vi "Write AcknowledgeMsg.vi"(8 "error in (no error)":errorcluster, 10 "AcknowledgeMsg.lvlib:AcknowledgeMsg.lvclass":refnum<class "CS++AcknowledgeMsg.lvclass">, 11 "AsynchReturnMsg in":refnum<class "CS++AsynchReturnMsg.lvclass">) -> (0 "error out":errorcluster, 3 "AsynchReturnMsg out":refnum<class "CS++AsynchReturnMsg.lvclass">)   [LabVIEW 2016, in "CS++AsynchReturnMsg.lvlib" / "CS++AsynchReturnMsg.lvclass"]
uses:
  CS++AsynchReturnMsg.lvclass
  CS++AcknowledgeMsg/CS++AcknowledgeMsg.lvclass
  CS++AsynchReturnMsg.lvclass/CS++AsynchReturnMsg.ctl
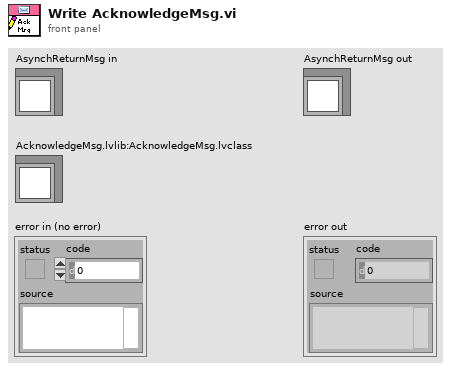
[diagram p1: front panel]
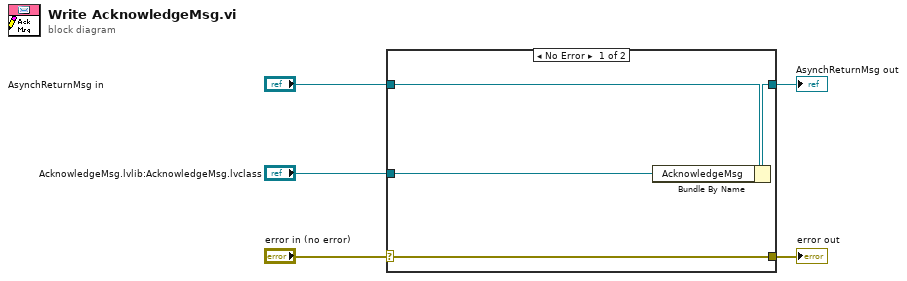
[diagram p0: block diagram]
diagram:
  n1 = case shown="No Error" "error in (no error)" {
    selector: "error in (no error)" -> [w9 w10]
    tunnel: [w9 w10] -> w4
    tunnel: [w7 w11] -> w2
    tunnel: "AsynchReturnMsg in" -> [w8 w11]
    tunnel: "AcknowledgeMsg.lvlib:AcknowledgeMsg.lvclass" -> [w6 _]
    frame No Error {
      n2 = Bundle By Name(cluster=w8, "AcknowledgeMsg"=w6) -> (w7:refnum<class "CS++AsynchReturnMsg.lvclass">)
    }
    frame Error {
    }
  }
  "error out" <- w4
  "AsynchReturnMsg out" <- w2
